vi "stop.vi"(8 "error in (no error)":errorcluster, 11 "TemperatureSensor in":refnum<class "TemperatureSensor.lvclass">) -> (0 "error out":errorcluster, 3 "TemperatureSensor out":refnum<class "TemperatureSensor.lvclass">)   [LabVIEW 2013, in "TemperatureSensor.lvclass"]
uses:
  TemperatureSensor.lvclass
  TemperatureSensor.lvclass/TemperatureSensor.ctl
  <userlib>/Common/SerialProtocols/SerialCommunicator/SerialCommunicator.lvclass
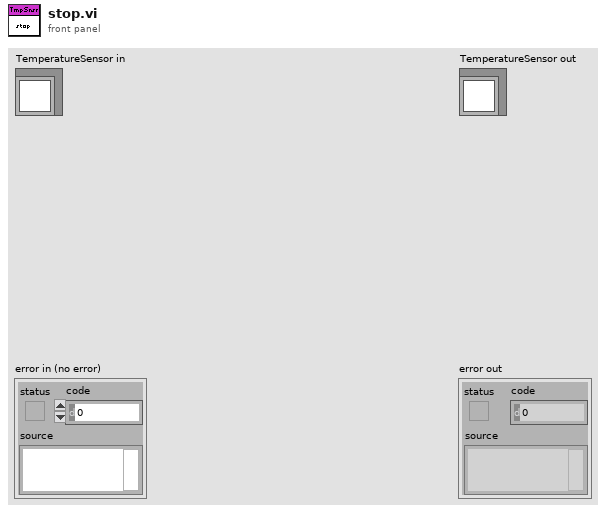
[diagram p1: front panel]
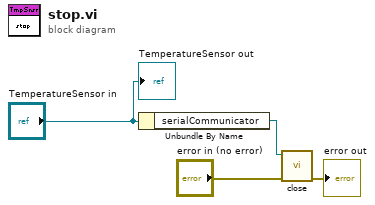
[diagram p0: block diagram]
diagram:
  n1 = Unbundle By Name("TemperatureSensor in") -> ("serialCommunicator"=w4:refnum<class "SerialCommunicator.lvclass">)
  n2 = call-dynamic "close.vi"("error in (no error)"="error in (no error)", "SerialCommunicator in"=w4) -> ("error out"=→"error out":errorcluster)  [unwired: 8 in, 1 out]
  "TemperatureSensor out" <- "TemperatureSensor in"
